vi "Camera Message Loop.vi"(8 "error in (no error)":errorcluster, 9 "Data Queue":refnum<queue>, 10 "Data Notifier":refnum<notifier>, 11 "Message Queues":T1) -> (0 "error out":errorcluster)   [LabVIEW 2015, in "Camera.lvlib"]
uses:
  Camera.lvlib
  support/Message Queue/All Message Queues.ctl
  support/Message Queue/Message Cluster.ctl
  <vilib>/vision/Image Controls.llb/IMAQ Image.ctl
  Camera Configuration.ctl
  Camera State.ctl
  Camera Loop State.ctl
  <vilib>/Utility/miscctls.llb/LVMinMaxIncTypeDef.ctl
  Acquisition Settings.ctl
  Live View State.ctl
  <vilib>/Utility/error.llb/Error Cluster From Error Code.vi
  <vilib>/ErrorRing/Error Ring.xnode
  support/Message Queue/Message Queue.lvlib
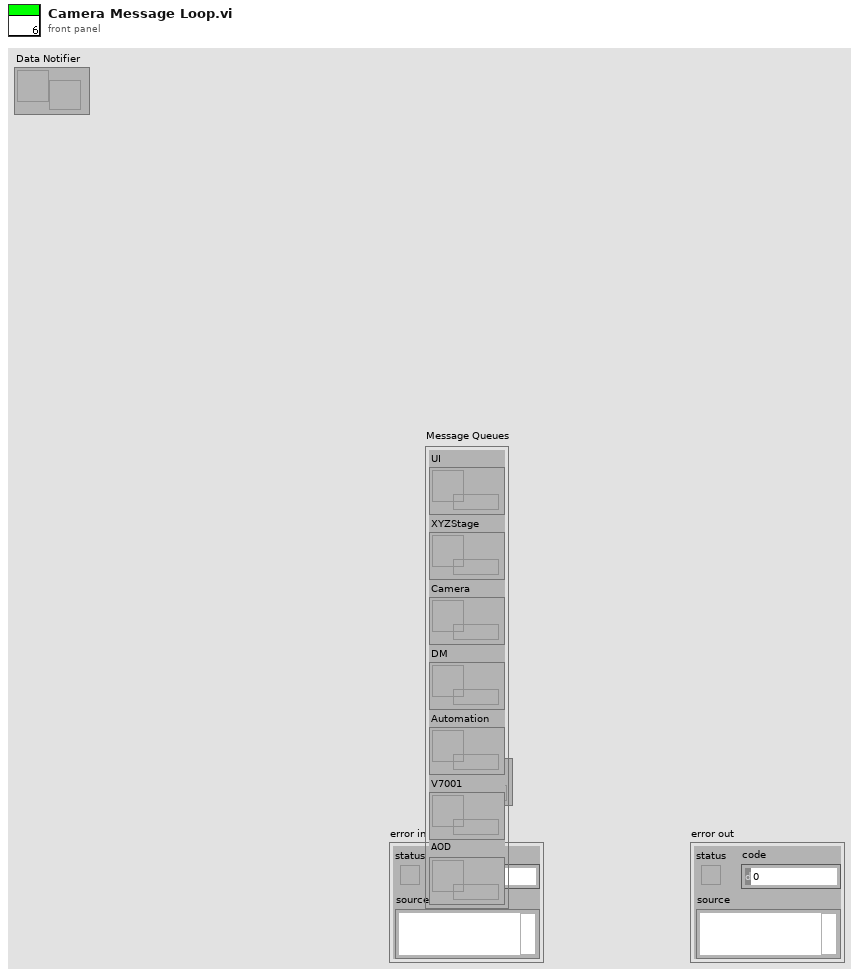
[diagram p1: front panel]
types:
  T1 = typedef "Message Queue.lvlib/All Message Queues.ctl" = cluster{"UI":refnum<queue>, "XYZStage":refnum<queue>, "Camera":refnum<queue>, "DM":refnum<queue>, "Automation":refnum<queue>, "V7001":refnum<queue>, "AOD":refnum<queue>}
  T2 = typedef "Camera.lvlib/Camera State.ctl" = cluster{"Camera State":T3, "Current Frame":i32, "Handle out":u32, "Camera Details":cluster{"Model":string, "Camera ID":string, "Firmware":string}, "Sub Region":cluster{"H Offset":cluster{"Value":i32, "Limits":T4}, "V Offset":cluster{"Value":i32, "Limits":T4}, "H Size":cluster{"Value":i32, "Limits":T4}, "V Size":cluster{"Value":i32, "Limits":T4}}, "Acquisition Settings":T5, "Live View State":T6}
  T3 = typedef "Camera.lvlib/Camera Loop State.ctl" = enum16{"Idle", "Live View", "Ready", "Acquiring"}
  T4 = typedef "LVMinMaxIncTypeDef.ctl" = cluster{"Minimum":dbl, "Maximum":dbl, "Increment":dbl}
  T5 = typedef "Camera.lvlib/Acquisition Settings.ctl" = cluster{"Save?":bool, "DCIMG Path":path, "Filename":string, "Total Frames":i32, "Sender":enum16{"UI", "Automation"}}
  T6 = typedef "Camera.lvlib/Live View State.ctl" = cluster{"Loop Counter":i32, "Time Of Latest Frame":u32, "Frame Count":u32, "FPS frames":dbl, "FPS Time":u32, "Current FPS":dbl}
  T7 = typedef "Camera.lvlib/Camera Configuration.ctl" = cluster{"Camera Index":u32}
  T8 = cluster{"Model":string, "Camera ID":string, "Firmware":string}
  T9 = typedef "IMAQ Image.ctl" = refnum<image>
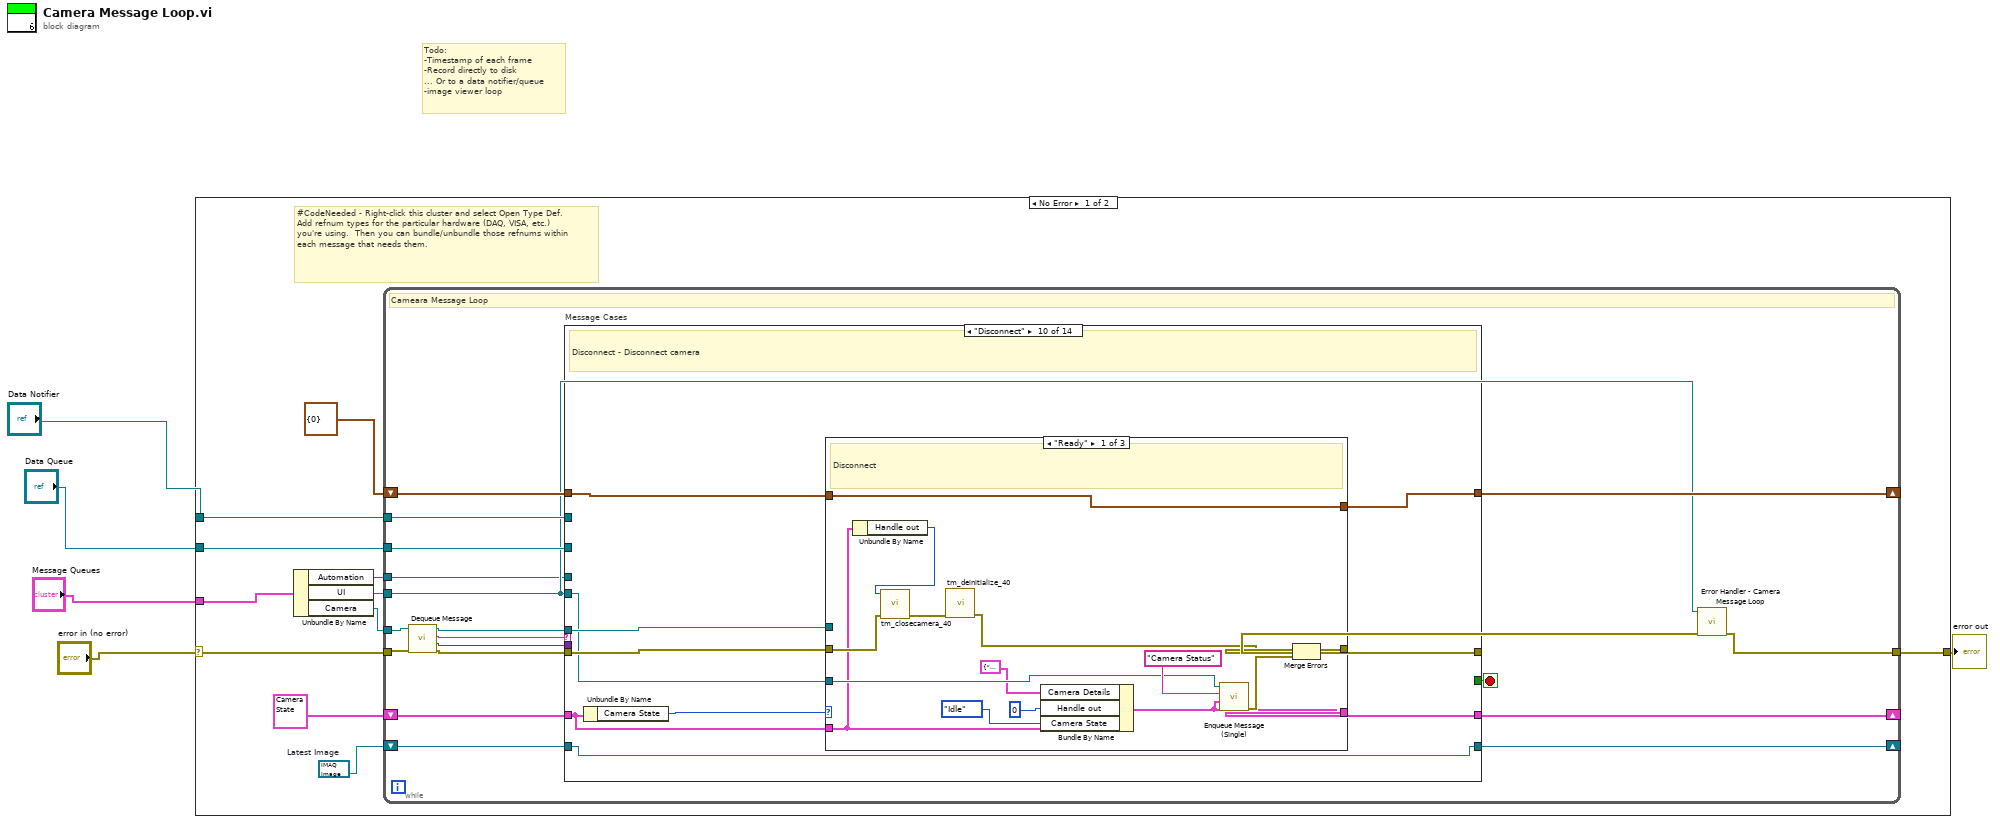
[diagram p0: block diagram]
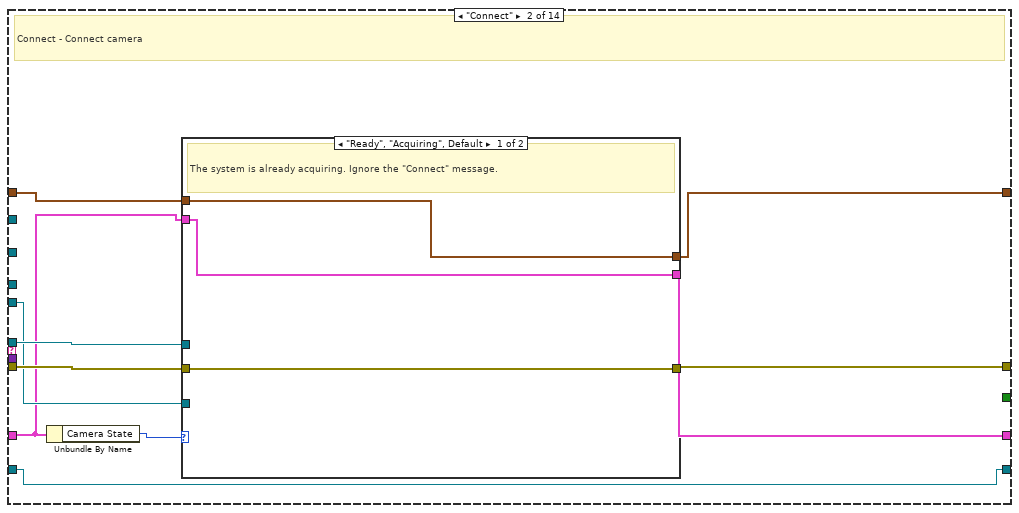
[diagram p3: hidden frame]
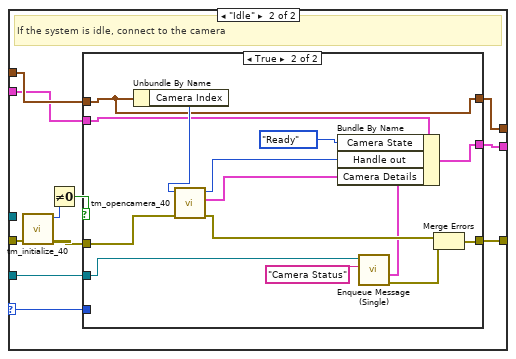
[diagram p4: hidden frame]
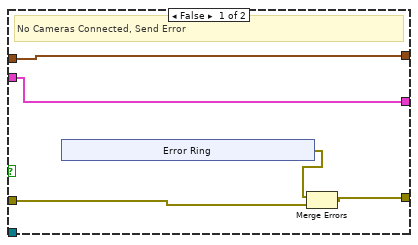
[diagram p5: hidden frame]
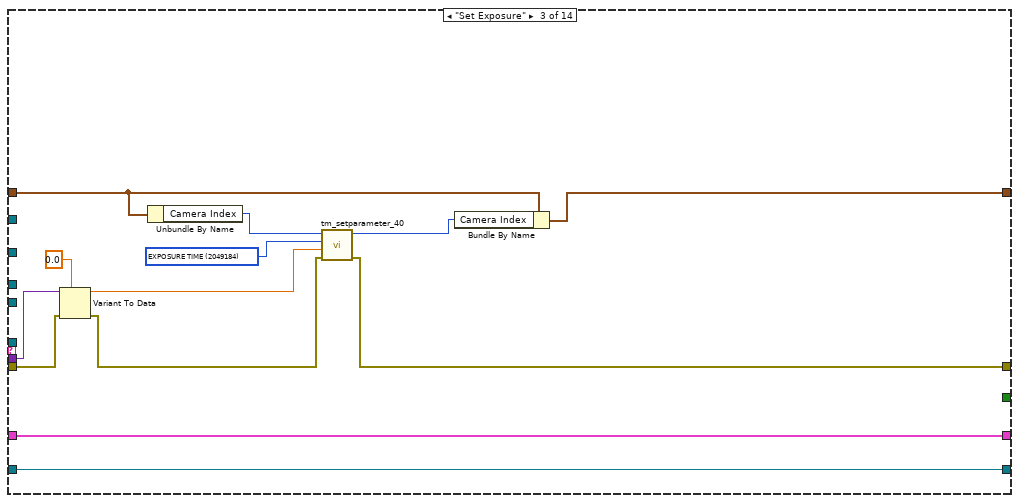
[diagram p6: hidden frame]
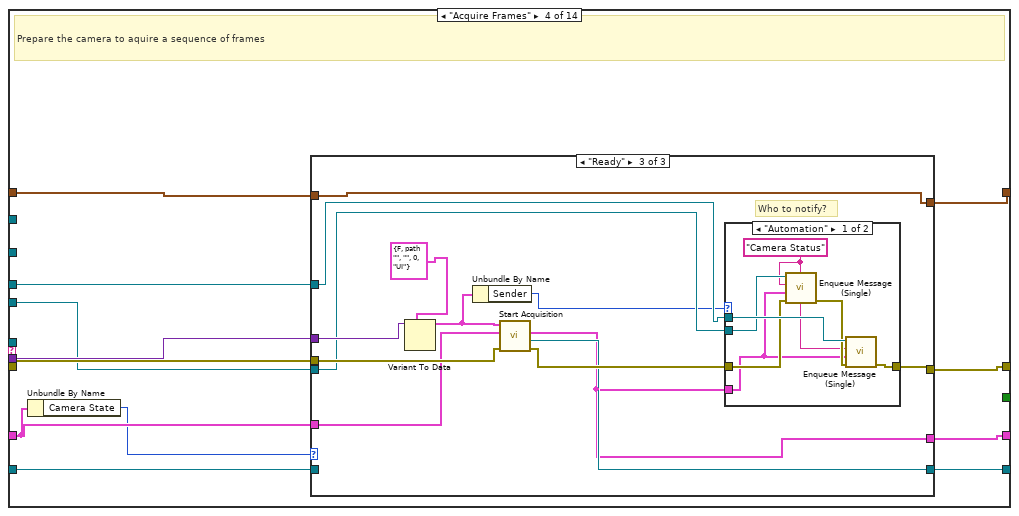
[diagram p7: hidden frame]
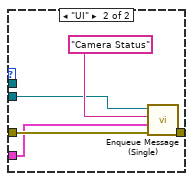
[diagram p10: hidden frame]
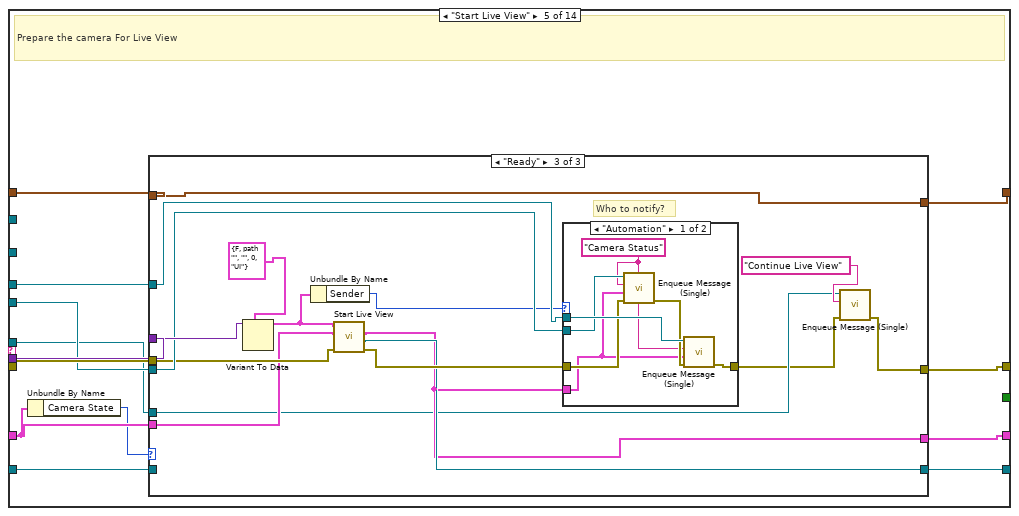
[diagram p11: hidden frame]
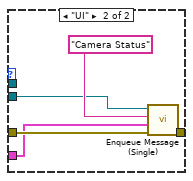
[diagram p14: hidden frame]
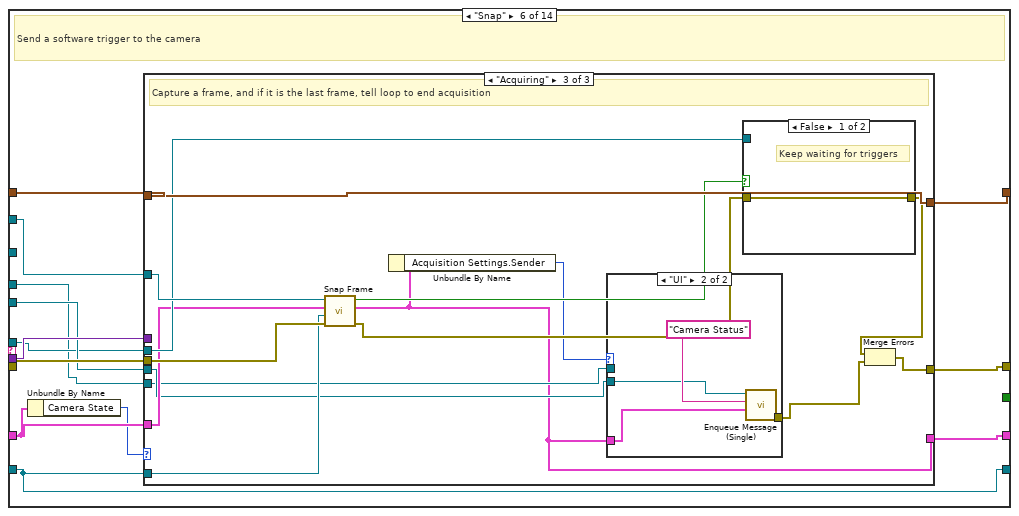
[diagram p15: hidden frame]
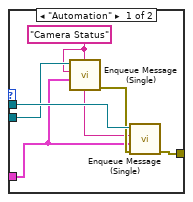
[diagram p18: hidden frame]
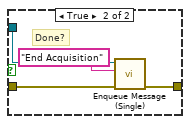
[diagram p19: hidden frame]
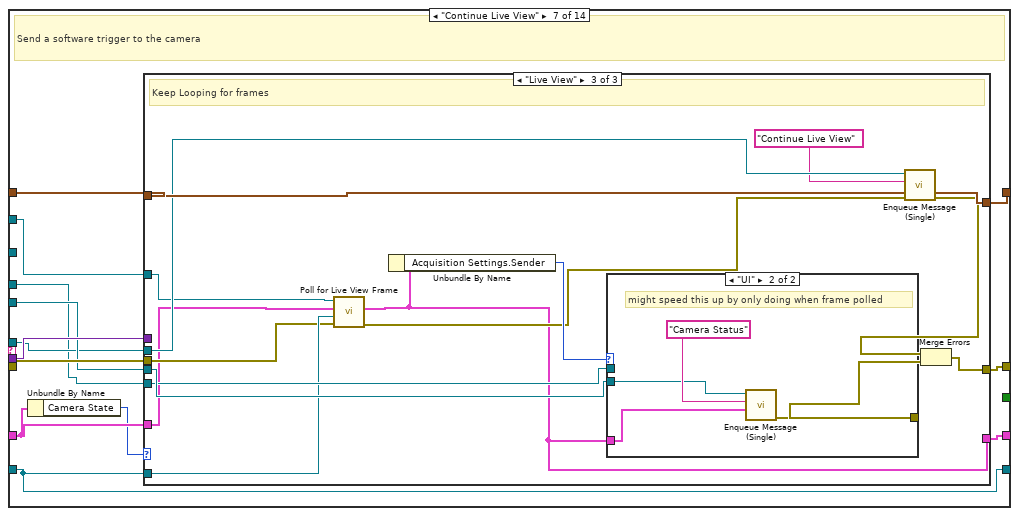
[diagram p20: hidden frame]
diagram:
  # "Todo:\n-Timestamp of each frame\n-Record directly to disk\n... Or to a data notifier/queue\n-image viewer loop"
  n1 = case shown="No Error" "error in (no error)" {
    selector: "error in (no error)" -> [w13 w437]
    tunnel: "Message Queues" -> [w16 _]
    tunnel: [w14 w437] -> w5
    tunnel: "Data Notifier" -> [w11 _]
    tunnel: "Data Queue" -> [w10 _]
    frame No Error {
      w7 = T9 refnum  # Latest Image
      # "#CodeNeeded - Right-click this cluster and select Open Type Def.  Add refnum types for the particular hardware (DAQ, VISA, etc.) you're using.  Then you can bundle/unbundle those refnums within each message that needs them."
      n2 = Unbundle By Name(w16) -> ("Automation"=w6:refnum<queue>, "UI"=w12:refnum<queue>, "Camera"=w15:refnum<queue>)
      n3 = while {
        tunnel: w15 -> [w28]
        shift-right: [w34] -> _
        shift-left: T7 {"Camera Index"=0} ("Hardware Configuration") -> [w35]
        tunnel: w12 -> [w20]
        tunnel: w11 -> [w32]
        tunnel: w10 -> [w31]
        shift-right: [w29] -> _
        shift-left: T2 {"Camera State"=enum."Idle", "Current Frame"=0, "Handle out"=0, "Camera Details"={"Model"="", "Camera ID"="", "Firmware"=""}, "Sub Region"={"H Offset"={"Value"=0, "Limits"={"Minimum"=0.0, "Maximum"=0.0, "Increment"=0.0}}, "V Offset"={"Value"=0, "Limits"={"Minimum"=0.0, "Maximum"=0.0, "Increment"=0.0}}, "H Size"={"Value"=0, "Limits"={"Minimum"=0.0, "Maximum"=0.0, "Increment"=0.0}}, "V Size"={"Value"=0, "Limits"={"Minimum"=0.0, "Maximum"=0.0, "Increment"=0.0}}}, "Acquisition Settings"={"Save?"=FALSE, "DCIMG Path"=path "", "Filename"="", "Total Frames"=0, "Sender"=enum."UI"}, "Live View State"={"Loop Counter"=0, "Time Of Latest Frame"=0, "Frame Count"=0, "FPS frames"=0.0, "FPS Time"=0, "Current FPS"=0.0}} ("Cluster") -> [w30]
        tunnel: w13 -> [w27]
        tunnel: [w22] -> w14
        shift-right: [w18] -> _
        shift-left: w7 -> [w19]
        tunnel: w6 -> [w17]
        stop <- w33 stop-if-true
        # "Cameara Message Loop"
        n4 = call "Dequeue Message.vi"("error in (no error)"=w27, "Message Queue"=w28) -> ("error out"=w23:errorcluster, "Message Data"=w24:variant, "Message"=w25:string, "dup Message Queue"=w26:refnum<queue>)  [unwired: 6 in]
        n5 = case "Message Cases" shown="\"Disconnect\"" w25 {
          selector: w25 -> [_ _ _ _ _ _ _ _ _ _ _ _ _ w426]
          tunnel: w26 -> [_ w46 _ _ w145 w197 w246 w288 w328 w374 w409 w414 _ _]
          tunnel: w23 -> [w39 w47 w93 w110 w156 w205 w254 w296 w336 w375 w407 w416 w424 _]
          tunnel: [w39 w49 w96 w106 w152 w201 w250 w292 w332 w377 w406 w418 w422 w427] -> w21
          tunnel: w35 -> [w37 w48 w89 w109 w155 w204 w253 w295 w335 w376 w411 w417 w423 w429]
          tunnel: [w37 w44 w88 w108 w154 w203 w252 w294 w334 w372 w411 w417 w423 w429] -> w34
          tunnel: [_ _ _ _ _ _ _ _ _ _ _ TRUE _ _] -> w33
          tunnel: w24 -> [_ _ w94 w111 w157 w206 w255 w297 w337 _ _ _ _ _]
          tunnel: w20 -> [_ w43 _ w107 w153 w202 w251 w293 w333 w371 _ _ _ _]
          tunnel: w32 -> [_ _ _ _ _ w195 w244 _ _ _ _ _ _ _]
          tunnel: w31 -> [_ _ _ _ _ _ _ _ _ _ _ _ _ _]
          tunnel: w30 -> [w38 w41 w99 w104 w150 w199 w248 w290 w330 w369 w410 w413 w421 w428]
          tunnel: [w38 w45 w99 w105 w151 w200 w249 w291 w331 w373 w410 w413 w421 w428] -> w29
          tunnel: w19 -> [w36 w40 w98 w102 w148 w196 w245 w287 w327 w368 w405 w412 w420 w425]
          tunnel: [w36 w40 w98 w103 w149 w196 w245 w287 w327 w368 w405 w412 w420 w425] -> w18
          tunnel: w17 -> [_ _ _ w101 w147 w194 w243 _ _ _ _ _ _ _]
          frame "Initialize" {
            # "Initialize  - Initialize is currently a no-op.  The hardware initialization takes place in the 'Start' message."
          }
          frame "Connect" {
            # "Connect - Connect camera"
            n6 = Unbundle By Name(w41) -> ("Camera State"=w42:T3)
            n7 = case shown="\"Ready\", \"Acquiring\", Default" w42 {
              selector: w42 -> [_ w55]
              tunnel: [w51 w63] -> w49
              tunnel: w48 -> [w52 w58]
              tunnel: w47 -> [w51 w62]
              tunnel: w46 -> [_ _]
              tunnel: [w52 w57] -> w44
              tunnel: [w50 w56] -> w45
              tunnel: w43 -> [_ w54]
              tunnel: w41 -> [w50 w53]
              frame "Ready", "Acquiring", Default {
                # "The system is already acquiring. Ignore the \"Connect\" message."
              }
              frame "Idle" {
                # "If the system is idle, connect to the camera"
                n8 = call <userlib>:"tm_initialize_40.vi"("error in (no error)"=w62) -> ("error out"=w61:errorcluster, "Number Of Cameras"=w59:u32)  [unwired: 7 in, 2 out]
                n9 = Not Equal To 0?(x=w59) -> (x != 0?=w60:bool)
                n10 = case shown="True" w60 {
                  tunnel: [w66 w86] -> w63
                  tunnel: w61 -> [w65 w85]
                  tunnel: w58 -> [w68 w75]
                  tunnel: [w68 w75] -> w57
                  tunnel: [w64 w78] -> w56
                  tunnel: w55 -> [_ _]
                  tunnel: w54 -> [_ w82]
                  tunnel: w53 -> [w64 w79]
                  frame False {
                    # "No Cameras Connected, Send Error"
                    n11 = xnode "Error Ring"() -> ("error out"=w67:errorcluster)
                    n12 = Merge Errors(w67, w65) -> (w66:errorcluster)
                  }
                  frame True {
                    n13 = Unbundle By Name(w75) -> ("Camera Index"=w84:u32)
                    n14 = call <userlib>:"tm_opencamera_40.vi"("error in (no error)"=w85, "Camera Index"=w84) -> ("error out"=w83:errorcluster, "Camera Details"=w76:T8, "Handle out"=w77:u32)  [unwired: 7 in]
                    n15 = Bundle By Name(cluster=w79, "Camera State"=Camera_Loop_State."Ready", "Handle out"=w77, "Camera Details"=w76) -> (w78:T2)
                    n16 = call "Enqueue Message (Single).vi"("Message Data"=w78, "Message"="Camera Status", "Message Queue"=w82) -> ("error out"=w80:errorcluster)  [unwired: 7 in, 1 out]
                    n17 = Merge Errors(w83, w80) -> (w86:errorcluster)
                  }
                }
              }
            }
          }
          frame "Set Exposure" {
            w95 = u32 2049184 items=["SENSOR MODE"=4212128, "READOUT SPEED"=4211872, "READOUT DIRECTION"=4211904, "TRIGGER GLOBAL EXPOSURE"=2049680, "TRIGGER DELAY"=1066480, "INTERNAL TRIGGER HANDLING"=1066496, "SYNC READOUT SYSTEM BLANK"=1066528, "SENSOR TEMPERATURE"=2115232, "SENSOR COOLER STATUS"=2115280, "EXPOSURE TIME"=2049184, "DEFECT CORRECT MODE"=4670368, "BINNING"=4215968, "INTERNAL LINE SPEED"=4226000, "INTERNAL LINE INTERVAL"=4226016, "NUMBER OF OUTPUT TRIGGER CONNECTOR"=1852320, "OUTPUT TRIGGER SOURCE[0]"=1852576, "OUTPUT TRIGGER SOURCE[1]"=1852832, "OUTPUT TRIGGER SOURCE[2]"=1853088, "OUTPUT TRIGGER POLARITY[0]"=1852592, "OUTPUT TRIGGER POLARITY[1]"=1852848, "OUTPUT TRIGGER POLARITY[2]"=1853104, "OUTPUT TRIGGER ACTIVE[0]"=1852608, "OUTPUT TRIGGER ACTIVE[1]"=1852864, "OUTPUT TRIGGER ACTIVE[2]"=1853120, "OUTPUT TRIGGER DELAY[0]"=1852624, "OUTPUT TRIGGER DELAY[1]"=1852880, "OUTPUT TRIGGER DELAY[2]"=1853136, "OUTPUT TRIGGER PERIOD[0]"=1852640, "OUTPUT TRIGGER PERIOD[1]"=1852896, "OUTPUT TRIGGER PERIOD[2]"=1853152, "OUTPUT TRIGGER KIND[0]"=1852656, "OUTPUT TRIGGER KIND[1]"=1852912, "OUTPUT TRIGGER KIND[2]"=1853168, "OUTPUT TRIGGER BASE SENSOR[0]"=1852672, "OUTPUT TRIGGER BASE SENSOR[1]"=1852928, "OUTPUT TRIGGER BASE SENSOR[2]"=1853184, "OUTPUT TRIGGER PRE HSYNC COUNT"=1852704] ("Parameter")
            n18 = Variant To Data(error in=w93, type=0.0 ("Value in"), Variant=w94) -> (data=w90:dbl, error out=w92:errorcluster)
            n19 = Unbundle By Name(w89) -> ("Camera Index"=w97:u32)
            n20 = call <userlib>:"tm_setparameter_40.vi"("error in (no error)"=w92, "Value in"=w90, "Parameter"=w95, "Handle in"=w97) -> ("error out"=w96:errorcluster, "Handle out"=w87:u32)  [unwired: 6 in]
            n21 = Bundle By Name(cluster=w89, "Camera Index"=w87) -> (w88:T7)
          }
          frame "Acquire Frames" {
            # "Prepare the camera to aquire a sequence of frames"
            n22 = Unbundle By Name(w104) -> ("Camera State"=w100:T3)
            n23 = case shown="\"Ready\"" w100 {
              tunnel: w111 -> [_ _ w132]
              tunnel: w110 -> [w114 w118 w129]
              tunnel: w109 -> [w115 w119 w130]
              tunnel: [w115 w119 w130] -> w108
              tunnel: w104 -> [w113 w117 w128]
              tunnel: w107 -> [_ _ w125]
              tunnel: [w114 w118 w131] -> w106
              tunnel: [w113 w117 w124] -> w105
              tunnel: [w112 w116 w126] -> w103
              tunnel: w102 -> [w112 w116 _]
              tunnel: w101 -> [_ _ w123]
              frame "Idle", Default {
                # "Not ready to acquire... do nothing"
              }
              frame "Acquiring" {
                # "Already acquiring, do nothing"
              }
              frame "Ready" {
                # "Who to notify?"
                n24 = Variant To Data(type=T5 {"Save?"=FALSE, "DCIMG Path"=path "", "Filename"="", "Total Frames"=0, "Sender"=enum."UI"} ("Acquisition Settings"), Variant=w132) -> (data=w122:T5)  [unwired: 1 in, 1 out]
                n25 = Unbundle By Name(w122) -> ("Sender"=w120:enum16{"UI", "Automation"})
                n26 = call "Start Acquisition.vi"("error in (no error)"=w129, "Camera State In"=w128, "Acquisition Settings"=w122) -> ("error out"=w127:errorcluster, "New Image Out"=w126:T9, "Camera State Out"=w124:T2)  [unwired: 6 in]
                n27 = case shown="\"Automation\"" w120 {
                  tunnel: [w139 w143] -> w131
                  tunnel: w127 -> [w137 w142]
                  tunnel: w125 -> [w135 w141]
                  tunnel: w124 -> [w133 w140]
                  tunnel: w123 -> [w138 _]
                  frame "Automation" {
                    w134 = "Camera Status" ("Message")
                    n28 = call "Enqueue Message (Single).vi"("error in (no error)"=w137, "Message Data"=w133, "Message"=w134, "Message Queue"=w135) -> ("error out"=w136:errorcluster)  [unwired: 6 in, 1 out]
                    n29 = call "Enqueue Message (Single).vi"("error in (no error)"=w136, "Message Data"=w133, "Message"=w134, "Message Queue"=w138) -> ("error out"=w139:errorcluster)  [unwired: 6 in, 1 out]
                  }
                  frame "UI" {
                    n30 = call "Enqueue Message (Single).vi"("error in (no error)"=w142, "Message Data"=w140, "Message"="Camera Status", "Message Queue"=w141) -> ("error out"=w143:errorcluster)  [unwired: 6 in, 1 out]
                  }
                }
              }
            }
          }
          frame "Start Live View" {
            # "Prepare the camera For Live View"
            n31 = Unbundle By Name(w150) -> ("Camera State"=w146:T3)
            n32 = case shown="\"Ready\"" w146 {
              tunnel: w157 -> [_ _ w181]
              tunnel: w156 -> [w160 w164 w174]
              tunnel: w155 -> [w161 w165 w180]
              tunnel: [w161 w165 w180] -> w154
              tunnel: w150 -> [w159 w163 w173]
              tunnel: w153 -> [_ _ w179]
              tunnel: [w160 w164 w166] -> w152
              tunnel: [w159 w163 w171] -> w151
              tunnel: [w158 w162 w172] -> w149
              tunnel: w148 -> [w158 w162 _]
              tunnel: w147 -> [_ _ w178]
              tunnel: w145 -> [_ _ w168]
              frame "Idle", Default {
                # "Not ready to acquire... do nothing"
              }
              frame "Acquiring" {
                # "Already acquiring, do nothing"
              }
              frame "Ready" {
                # "Who to notify?"
                n33 = Variant To Data(type=T5 {"Save?"=FALSE, "DCIMG Path"=path "", "Filename"="", "Total Frames"=0, "Sender"=enum."UI"} ("Acquisition Settings"), Variant=w181) -> (data=w170:T5)  [unwired: 1 in, 1 out]
                n34 = Unbundle By Name(w170) -> ("Sender"=w176:enum16{"UI", "Automation"})
                n35 = call "Start Live View.vi"("error in (no error)"=w174, "Camera State In"=w173, "Acquisition Settings"=w170) -> ("error out"=w175:errorcluster, "New Image Out"=w172:T9, "Camera State Out"=w171:T2)  [unwired: 6 in]
                n36 = case shown="\"Automation\"" w176 {
                  tunnel: [w188 w192] -> w167
                  tunnel: w175 -> [w186 w191]
                  tunnel: w179 -> [w184 w190]
                  tunnel: w171 -> [w182 w189]
                  tunnel: w178 -> [w187 _]
                  frame "Automation" {
                    w183 = "Camera Status" ("Message")
                    n37 = call "Enqueue Message (Single).vi"("error in (no error)"=w186, "Message Data"=w182, "Message"=w183, "Message Queue"=w184) -> ("error out"=w185:errorcluster)  [unwired: 6 in, 1 out]
                    n38 = call "Enqueue Message (Single).vi"("error in (no error)"=w185, "Message Data"=w182, "Message"=w183, "Message Queue"=w187) -> ("error out"=w188:errorcluster)  [unwired: 6 in, 1 out]
                  }
                  frame "UI" {
                    n39 = call "Enqueue Message (Single).vi"("error in (no error)"=w191, "Message Data"=w189, "Message"="Camera Status", "Message Queue"=w190) -> ("error out"=w192:errorcluster)  [unwired: 6 in, 1 out]
                  }
                }
                n40 = call "Enqueue Message (Single).vi"("error in (no error)"=w167, "Message"="Continue Live View", "Message Queue"=w168) -> ("error out"=w166:errorcluster)  [unwired: 7 in, 1 out]
              }
            }
          }
          frame "Snap" {
            # "Send a software trigger to the camera"
            n41 = Unbundle By Name(w199) -> ("Camera State"=w198:T3)
            n42 = case shown="\"Acquiring\"" w198 {
              tunnel: w206 -> [_ _ _]
              tunnel: w205 -> [w208 w211 w223]
              tunnel: w204 -> [w209 w212 w227]
              tunnel: [w209 w212 w227] -> w203
              tunnel: w199 -> [w207 w210 w218]
              tunnel: w202 -> [_ _ w216]
              tunnel: [w208 w211 w226] -> w201
              tunnel: [w207 w210 w214] -> w200
              tunnel: w197 -> [_ _ w220]
              tunnel: w196 -> [_ _ w221]
              tunnel: w195 -> [_ _ w224]
              tunnel: w194 -> [_ _ w215]
              frame "Idle", Default {
                # "Not ready to acquire... do nothing"
              }
              frame "Ready" {
                # "Ready state, not acquiring, do nothing"
              }
              frame "Acquiring" {
                # "Capture a frame, and if it is the last frame, tell loop to end acquisition"
                n43 = call "Snap Frame.vi"("error in (no error)"=w223, "Imaq Image pointer"=w221, "Camera State In"=w218, "Image Data Notifier"=w224) -> ("error in (no error) 2"=w219:errorcluster, "Camera State Out"=w214:T2, "Done?"=w222:bool)  [unwired: 4 in, 1 out]
                n44 = Unbundle By Name(w214) -> ("Acquisition Settings.Sender"=w213:enum16{"UI", "Automation"})
                n45 = case shown="\"UI\"" w213 {
                  tunnel: [w233 w236] -> w217
                  tunnel: w216 -> [w230 w235]
                  tunnel: w214 -> [w228 w234]
                  tunnel: w215 -> [w232 _]
                  frame "Automation" {
                    w229 = "Camera Status" ("Message")
                    n46 = call "Enqueue Message (Single).vi"("Message Data"=w228, "Message"=w229, "Message Queue"=w230) -> ("error out"=w231:errorcluster)  [unwired: 7 in, 1 out]
                    n47 = call "Enqueue Message (Single).vi"("error in (no error)"=w231, "Message Data"=w228, "Message"=w229, "Message Queue"=w232) -> ("error out"=w233:errorcluster)  [unwired: 6 in, 1 out]
                  }
                  frame "UI" {
                    n48 = call "Enqueue Message (Single).vi"("Message Data"=w234, "Message"="Camera Status", "Message Queue"=w235) -> ("error out"=w236:errorcluster)  [unwired: 7 in, 1 out]
                  }
                }
                n49 = case shown="False" w222 {
                  tunnel: w220 -> [_ w242]
                  tunnel: [w238 w240] -> w225
                  tunnel: w219 -> [w238 w239]
                  frame False {
                    # "Keep waiting for triggers"
                  }
                  frame True {
                    # "Done?"
                    n50 = call "Enqueue Message (Single).vi"("error in (no error)"=w239, "Message"="End Acquisition", "Message Queue"=w242) -> ("error out"=w240:errorcluster)  [unwired: 7 in, 1 out]
                  }
                }
                n51 = Merge Errors(w225, w217) -> (w226:errorcluster)
              }
            }
          }
          frame "Continue Live View" {
            # "Send a software trigger to the camera"
            n52 = Unbundle By Name(w248) -> ("Camera State"=w247:T3)
            n53 = case shown="\"Live View\"" w247 {
              tunnel: w255 -> [_ _ _]
              tunnel: w254 -> [w257 w260 w266]
              tunnel: w253 -> [w258 w261 w276]
              tunnel: [w258 w261 w276] -> w252
              tunnel: w248 -> [w256 w259 w263]
              tunnel: w251 -> [_ _ w271]
              tunnel: [w257 w260 w275] -> w250
              tunnel: [w256 w259 w264] -> w249
              tunnel: w246 -> [_ _ w273]
              tunnel: w245 -> [_ _ w267]
              tunnel: w244 -> [_ _ w268]
              tunnel: w243 -> [_ _ w270]
              frame "Idle", Default {
                # "Not ready to acquire... do nothing"
              }
              frame "Ready" {
                # "Ready state, not acquiring, do nothing"
              }
              frame "Live View" {
                # "Keep Looping for frames"
                n54 = call "Poll for Live View Frame.vi"("error in (no error)"=w266, "Imaq Image pointer"=w267, "Camera State In"=w263, "Image Data Notifier"=w268) -> ("error in (no error) 2"=w265:errorcluster, "Camera State Out"=w264:T2)  [unwired: 5 in, 1 out]
                n55 = Unbundle By Name(w264) -> ("Acquisition Settings.Sender"=w269:enum16{"UI", "Automation"})
                n56 = case shown="\"UI\"" w269 {
                  tunnel: [w282 w285] -> w272
                  tunnel: w271 -> [w279 w284]
                  tunnel: w264 -> [w277 w283]
                  tunnel: w270 -> [w281 _]
                  frame "Automation" {
                    w278 = "Camera Status" ("Message")
                    n57 = call "Enqueue Message (Single).vi"("Message Data"=w277, "Message"=w278, "Message Queue"=w279) -> ("error out"=w280:errorcluster)  [unwired: 7 in, 1 out]
                    n58 = call "Enqueue Message (Single).vi"("error in (no error)"=w280, "Message Data"=w277, "Message"=w278, "Message Queue"=w281) -> ("error out"=w282:errorcluster)  [unwired: 6 in, 1 out]
                  }
                  frame "UI" {
                    # "might speed this up by only doing when frame polled"
                    n59 = call "Enqueue Message (Single).vi"("Message Data"=w283, "Message"="Camera Status", "Message Queue"=w284) -> ("error out"=w285:errorcluster)  [unwired: 7 in, 1 out]
                  }
                }
                n60 = call "Enqueue Message (Single).vi"("error in (no error)"=w265, "Message"="Continue Live View", "Message Queue"=w273) -> ("error out"=w274:errorcluster)  [unwired: 7 in, 1 out]
                n61 = Merge Errors(w274, w272) -> (w275:errorcluster)
              }
            }
          }
          frame "End Acquisition" {
            # "Send a software trigger to the camera"
            n62 = Unbundle By Name(w290) -> ("Camera State"=w289:T3)
            n63 = case shown="\"Acquiring\"" w289 {
              tunnel: w297 -> [_ _ _]
              tunnel: w296 -> [w299 w302 w314]
              tunnel: w295 -> [w300 w303 w320]
              tunnel: [w300 w303 w320] -> w294
              tunnel: w290 -> [w298 w301 w315]
              tunnel: w293 -> [_ _ w312]
              tunnel: [w299 w302 w316] -> w292
              tunnel: [w298 w301 w310] -> w291
              tunnel: w288 -> [_ _ _]
              frame "Idle", Default {
                # "Not ready to acquire... do nothing"
              }
              frame "Ready" {
                # "Ready state, not acquiring, do nothing"
              }
              frame "Acquiring" {
                # "Capture a frame, and if it is the last frame, tell loop to end acquisition"
                n64 = Unbundle By Name(w315) -> ("Handle out"=w319:u32, "Acquisition Settings.Save?"=w308:bool)
                n65 = call <userlib>:"tm_stopcapture_40.vi"("error in (no error)"=w314, "Handle in"=w319) -> ("error out"=w307:errorcluster, "Handle out"=w304:u32)  [unwired: 8 in]
                n66 = case shown="True" w308 {
                  tunnel: w307 -> [w322 w326]
                  tunnel: [w322 w325] -> w306
                  tunnel: [w321 w324] -> w305
                  tunnel: w304 -> [w321 w323]
                  frame False {
                  }
                  frame True {
                    n67 = call <userlib>:"tm_stoprecorder_40.vi"("error in (no error)"=w326, "Handle in"=w323) -> ("error out"=w325:errorcluster, "Handle out"=w324:u32)  [unwired: 8 in]
                  }
                }
                n68 = call <userlib>:"tm_unpreparecapture_40.vi"("error in (no error)"=w306, "Handle in"=w305) -> ("error out"=w313:errorcluster, "Handle out"=w318:u32)  [unwired: 8 in]
                n69 = Bundle By Name(cluster=w315, "Camera State"=Camera_Loop_State."Ready", "Handle out"=w318) -> (w310:T2)
                n70 = call "Enqueue Message (Single).vi"("error in (no error)"=w313, "Message Data"=w310, "Message"="Camera Status", "Message Queue"=w312) -> ("error out"=w309:errorcluster)  [unwired: 6 in, 1 out]
                n71 = Merge Errors(w309) -> (w316:errorcluster)
              }
            }
          }
          frame "Stop Live View" {
            # "Send a software trigger to the camera"
            n72 = Unbundle By Name(w330) -> ("Camera State"=w329:T3)
            n73 = case shown="\"Live View\"" w329 {
              tunnel: w337 -> [_ _ _]
              tunnel: w336 -> [w339 w342 w355]
              tunnel: w335 -> [w340 w343 w361]
              tunnel: [w340 w343 w361] -> w334
              tunnel: w330 -> [w338 w341 w356]
              tunnel: w333 -> [_ _ w353]
              tunnel: [w339 w342 w357] -> w332
              tunnel: [w338 w341 w351] -> w331
              tunnel: w328 -> [_ _ _]
              frame "Idle", Default {
                # "Not ready to acquire... do nothing"
              }
              frame "Ready" {
                # "Ready state, not acquiring, do nothing"
              }
              frame "Live View" {
                # "Stop Live View mode, put back into Ready state"
                n74 = Unbundle By Name(w356) -> ("Handle out"=w360:u32)
                n75 = call <userlib>:"tm_stopcapture_40.vi"("error in (no error)"=w355, "Handle in"=w360) -> ("error out"=w349:errorcluster, "Handle out"=w346:u32)  [unwired: 8 in]
                n76 = case shown="False" FALSE {
                  tunnel: w349 -> [w363 w367]
                  tunnel: [w363 w366] -> w348
                  tunnel: [w362 w365] -> w347
                  tunnel: w346 -> [w362 w364]
                  frame False {
                  }
                  frame True {
                    n77 = call <userlib>:"tm_stoprecorder_40.vi"("error in (no error)"=w367, "Handle in"=w364) -> ("error out"=w366:errorcluster, "Handle out"=w365:u32)  [unwired: 8 in]
                  }
                }
                n78 = call <userlib>:"tm_unpreparecapture_40.vi"("error in (no error)"=w348, "Handle in"=w347) -> ("error out"=w354:errorcluster, "Handle out"=w359:u32)  [unwired: 8 in]
                n79 = Bundle By Name(cluster=w356, "Camera State"=Camera_Loop_State."Ready", "Handle out"=w359, "Live View State"=T6 {"Loop Counter"=0, "Time Of Latest Frame"=0, "Frame Count"=0, "FPS frames"=0.0, "FPS Time"=0, "Current FPS"=0.0}) -> (w351:T2)
                n80 = call "Enqueue Message (Single).vi"("error in (no error)"=w354, "Message Data"=w351, "Message"="Camera Status", "Message Queue"=w353) -> ("error out"=w350:errorcluster)  [unwired: 6 in, 1 out]
                n81 = Merge Errors(w350) -> (w357:errorcluster)
              }
            }
          }
          frame "Disconnect" {
            # "Disconnect - Disconnect camera"
            n82 = Unbundle By Name(w369) -> ("Camera State"=w370:T3)
            n83 = case shown="\"Ready\"" w370 {
              tunnel: [w386 w399 w403] -> w377
              tunnel: w376 -> [w381 w401 w404]
              tunnel: w375 -> [w390 w393 w403]
              tunnel: w374 -> [_ w397 _]
              tunnel: [w381 w401 w404] -> w372
              tunnel: [w383 w394 w402] -> w373
              tunnel: w371 -> [w387 _ _]
              tunnel: w369 -> [w380 w394 w402]
              frame "Ready" {
                # "Disconnect"
                n84 = Unbundle By Name(w380) -> ("Handle out"=w391:u32)
                n85 = call <userlib>:"tm_closecamera_40.vi"("error in (no error)"=w390, "Handle in"=w391) -> ("error out"=w389:errorcluster)  [unwired: 9 in]
                n86 = call <userlib>:"tm_deinitialize_40.vi"("error in (no error)"=w389) -> ("error out"=w385:errorcluster)  [unwired: 10 in]
                n87 = Bundle By Name(cluster=w380, "Camera Details"=T8 {"Model"="", "Camera ID"="", "Firmware"=""}, "Handle out"=u32 0, "Camera State"=Camera_Loop_State."Idle") -> (w383:T2)
                n88 = call "Enqueue Message (Single).vi"("Message Data"=w383, "Message"="Camera Status", "Message Queue"=w387) -> ("error out"=w384:errorcluster)  [unwired: 7 in, 1 out]
                n89 = Merge Errors(w385, w384) -> (w386:errorcluster)
              }
              frame "Acquiring" {
                # "If stopping in the middle of acquisition, stop and unprep first"
                n90 = call "Enqueue Message (Single).vi"("error in (no error)"=w393, "Message"="End Acquisition", "Message Queue"=w397) -> ("error out"=w395:errorcluster, "dup Message Queue"=w396:refnum<queue>)  [unwired: 7 in]
                n91 = call "Enqueue Message (Single).vi"("error in (no error)"=w395, "Message"="Disconnect", "Message Queue"=w396) -> ("error out"=w398:errorcluster)  [unwired: 7 in, 1 out]
                n92 = Merge Errors(w398) -> (w399:errorcluster)
              }
              frame "Idle", Default {
                # "If the system is idle, do nothing"
              }
            }
          }
          frame "Stop" {
            n93 = call "Enqueue Message (Single).vi"("error in (no error)"=w407, "Message"="Disconnect", "Message Queue"=w409) -> ("error out"=w406:errorcluster)  [unwired: 7 in, 1 out]
          }
          frame "Exit" {
            # "Release the Acquisition queue reference"
            # "Stop the VI"
            # "Exit - Send the Exit message to the UI Message Handler."
            n94 = Release Queue(queue=w414, error in (no error)=w416) -> (error out=w415:errorcluster)  [unwired: 1 in, 2 out]
            n95 = Merge Errors(w415) -> (w418:errorcluster)
          }
          frame "---Copy This Frame---" {
            # "Duplicate this frame when creating new messages.  Change this comment in the duplicated frame to describe this message."
            n96 = Merge Errors(w424) -> (w422:errorcluster)
          }
          frame Default {
            # "'Default' case only runs if there is a message that isn't defined in any of the other cases.  Output a programming error."
            n97 = xnode "Error Ring"("parameter 0"=w426) -> ("error out"=w427:errorcluster)
          }
        }
        n98 = call "Error Handler - Camera Message Loop.vi"("error in (no error)"=w21, "Message Queue"=w20) -> ("dup error in"=w22:errorcluster)  [unwired: 8 in, 1 out]
      }
    }
    frame Error {
    }
  }
  "error out" <- w5
